vi "Encoder Raw to Inches.vi"(11 "Raw Sensor Units":i32) -> (3 "Scaled Units (in.)":dbl)   [LabVIEW 2018]
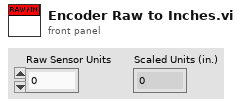
[diagram p1: front panel]
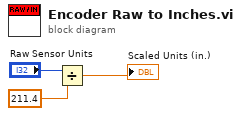
[diagram p0: block diagram]
diagram:
  n1 = Divide(x="Raw Sensor Units", y=211.4) -> (x/y=→"Scaled Units (in.)":dbl)
